vi "PI control (SubVI).vi"(0 "SetPoint":fxp<+/-,20,5>, 5 "Feedback":fxp<+/-,20,5>, 7 "Clock":fxp<+,32,32>, 9 "I":fxp<+/-,20,5>, 11 "P":fxp<+/-,20,5>, 12 "Initial I":fxp<+/-,20,5>, 13 "Lower Limit":fxp<+/-,64,29>, 14 "Upper Limit in":fxp<+/-,64,29>) -> (8 "Output":fxp<+/-,64,29>)   [LabVIEW 2017]
uses:
  <vilib>/rvi/FXPMathLib/FxpDiv/subVIs/nifxpmath_Div_SimConfig.ctl
  <vilib>/rvi/FXPMathLib/FxpDiv/simVIs/DllFxpDivTemp_sub.vi
  <vilib>/rvi/FXPMathLib/FxpDiv/XNode/nifxpmath_Div.xnode
  <vilib>/rvi/FXPMathLib/FxpSub/XNode/nifxpmath_Sub.xnode
  <vilib>/rvi/FXPMathLib/FxpMul/XNode/nifxpmath_Multiplier.xnode
  <vilib>/rvi/FXPMathLib/FxpAdd/XNode/nifxpmath_Add.xnode
  <vilib>/rvi/FXPMathLib/sim/FxpSim.dll
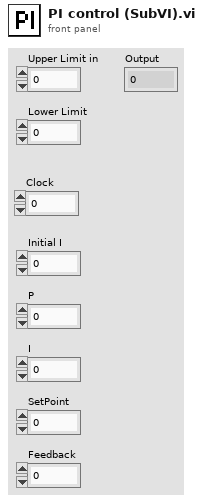
[diagram p1: front panel]
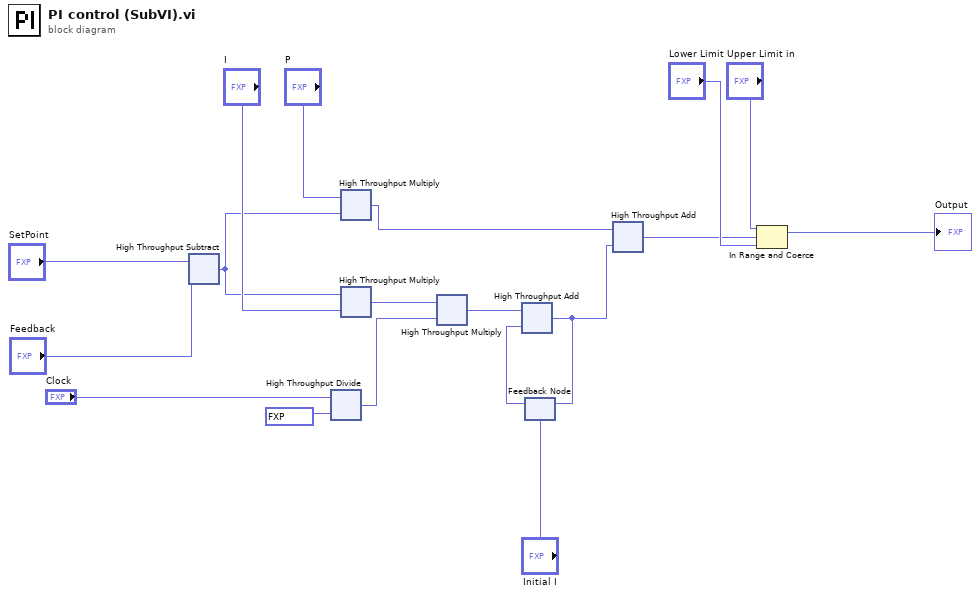
[diagram p0: block diagram]
diagram:
  n1 = xnode ("High Throughput Subtract")("x"="SetPoint", "y"="Feedback") -> ("x-y"=w9:fxp<+/-,64,16>)
  n2 = xnode "High Throughput Divide"("x"="Clock", "y"=fxp<+,14,20> 1000000.0) -> ("x/y"=w2:fxp<+,64,30>)
  n3 = xnode ("High Throughput Multiply")("x"="P", "y"=w9) -> ("x*y"=w5:fxp<+/-,64,27>)
  n4 = xnode ("High Throughput Multiply")("x"=w9, "y"="I") -> ("x*y"=w8:fxp<+/-,64,28>)
  n5 = xnode ("High Throughput Multiply")("x"=w8, "y"=w2) -> ("x*y"=w7:fxp<+/-,64,39>)
  n6 = feedback #1("Initial I") -> (w6:fxp<+/-,64,28>)
  n7 = xnode ("High Throughput Add")("x"=w7, "y"=w6) -> ("x+y"=w4:fxp<+/-,64,28>)
  n8 = feedback-in #1(w4) -> ()
  n9 = xnode ("High Throughput Add")("x"=w5, "y"=w4) -> ("x+y"=w3:fxp<+/-,64,29>)
  n10 = In Range and Coerce(upper limit="Upper Limit in", x=w3, lower limit="Lower Limit") -> (coerced(x)=→"Output":fxp<+/-,64,29>)  [unwired: 1 out]
